vi "Delete Event DVR.vi"(8 "error in (no error)":errorcluster, 11 "Event DVR in":refnum<data-value>) -> (0 "error out":errorcluster, 3 "Event out":refnum<class "Event.lvclass">)   [LabVIEW 2015, in "MDSplus.lvlib" / "Event.lvclass"]
uses:
  Event.lvclass
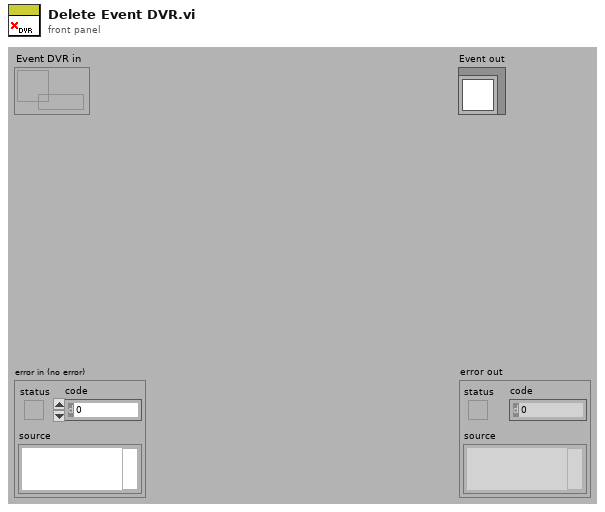
[diagram p1: front panel]
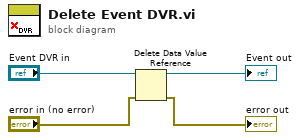
[diagram p0: block diagram]
diagram:
  n1 = Delete Data Value Reference(data value reference="Event DVR in", error in="error in (no error)") -> (data value=→"Event out":refnum<class "Event.lvclass">, error out=→"error out":errorcluster)
